vi "FTCGlobals.vi"(2 "Write?":bool, 4 "Write Globals":T1) -> (1 "Read Globals":T1)   [LabVIEW 2012, in "FTC.lvlib"]
uses:
  FTC.lvlib
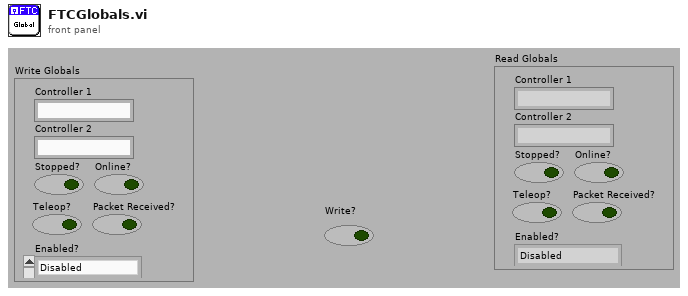
[diagram p1: front panel]
types:
  T1 = cluster{"Controller 1":string, "Controller 2":string, "Stopped?":bool, "Online?":bool, "Packet Received?":bool, "Teleop?":bool, "Enabled?":enum16{"Disabled", "Enabled"}}
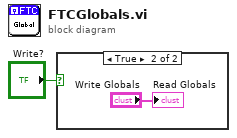
[diagram p0: block diagram]
diagram:
  n1 = case shown="True" "Write?" {
    frame False {
    }
    frame True {
      "Read Globals" <- "Write Globals"
    }
  }
